vi "Build_from_Wizard.vi"(8 "error in (no error)":errorcluster, 9 "programmatic":bool, 10 "preview":bool, 11 "Class in":refnum<class "Installer.lvclass">) -> (0 "error out":errorcluster, 3 "Class out":refnum<class "Installer.lvclass">)   [LabVIEW 2020, in "Installer.lvclass"]
uses:
  <vilib>/AppBuilder/IB_Classes/Installer/Installer.lvclass
  <vilib>/AppBuilder/IB_Classes/Installer/Installer.lvclass/Installer.ctl
  <resource>/Framework/Providers/API/mxLvBuildError.ctl
  <resource>/Framework/Providers/Common/provcom_ProgressBar_Events.ctl
  <resource>/Framework/Providers/Common/provcom_StringGlobals.vi
  <resource>/Framework/Providers/Common/provcom_ProgressBar_Dialog_Text.ctl
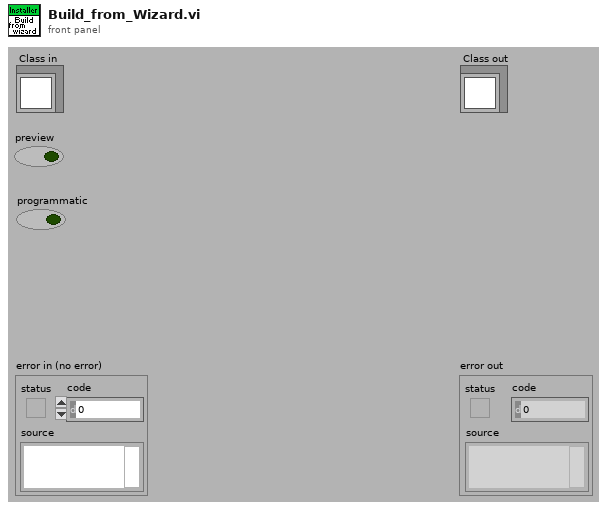
[diagram p1: front panel]
types:
  T1 = typedef "provcom_ProgressBar_Events.ctl" = cluster{"newJob":refnum<user-event>, "newItem":refnum<user-event>, "errorMsg":T2, "cancel":refnum<user-event>}
  T2 = typedef "mxLvBuildError.ctl" = refnum<user-event>
  T3 = typedef "provcom_ProgressBar_Dialog_Text.ctl" = cluster{"Operation action label":string, "Window title":string, "Expand text":string}
  T4 = typedef "mxLvBuildNewJob.ctl" = refnum<user-event>
  T5 = typedef "mxLvBuildNewItem.ctl" = refnum<user-event>
  T6 = typedef "mxLvBuildCancel.ctl" = refnum<user-event>
  T7 = typedef "ItemRef.ctl" = u64
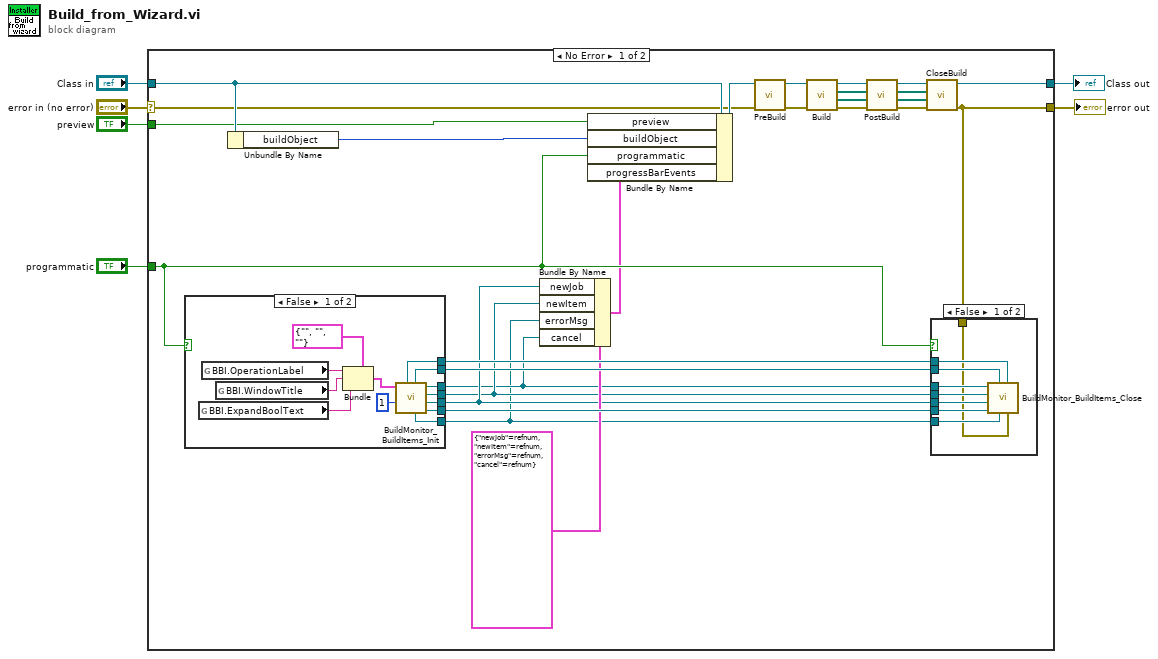
[diagram p0: block diagram]
diagram:
  n1 = case shown="No Error" "error in (no error)" {
    selector: "error in (no error)" -> [w7 w56]
    tunnel: [w14 w56] -> w5
    tunnel: [w20 w55] -> w3
    tunnel: "Class in" -> [w30 w55]
    tunnel: "preview" -> [w10 _]
    tunnel: "programmatic" -> [w9 _]
    frame No Error {
      n2 = case shown="False" w9 {
        tunnel: [w54 _] -> w33
        tunnel: [w53 _] -> w32
        tunnel: [w52 _] -> w31
        tunnel: [w51 _] -> w16
        tunnel: [w50 _] -> w17
        tunnel: [w49 _] -> w18
        tunnel: [w48 _] -> w15
        frame False {
          n3 = global read "provcom_StringGlobals.vi" "BBI.ExpandBoolText"() -> (w42:string)
          n4 = global read "provcom_StringGlobals.vi" "BBI.OperationLabel"() -> (w44:string)
          n5 = global read "provcom_StringGlobals.vi" "BBI.WindowTitle"() -> (w43:string)
          n6 = Bundle(cluster=T3 {"Operation action label"="", "Window title"="", "Expand text"=""} ("progressBar_DialogText"), "Operation action label"=w44, "Window title"=w43, "Expand text"=w42) -> (w45:T3)
          n7 = call <resource>:"BuildMonitor_BuildItems_Init.vi"("NumOfJobs"=u16 1, "progressBar_DialogText"=w45) -> ("Complete"=w54:refnum<user-event>, "NewJob"=w49:T4, "NewItem"=w50:T5, "Cancel event"=w51:T6, "Error event"=w48:T2, "ErrorOpenEvent"=w53:refnum<user-event>, "ErrorCloseEvent"=w52:refnum<user-event>)  [unwired: 3 in]
        }
        frame True {
        }
      }
      n8 = Unbundle By Name(w30) -> ("buildObject"=w13:T7)
      n9 = Bundle By Name(cluster=T1 {"newJob"=refnum, "newItem"=refnum, "errorMsg"=refnum, "cancel"=refnum} ("progressBarEvents"), "newJob"=w18, "newItem"=w17, "errorMsg"=w15, "cancel"=w16) -> (w8:T1)
      n10 = Bundle By Name(cluster=w30, "preview"=w10, "buildObject"=w13, "programmatic"=w9, "progressBarEvents"=w8) -> (w21:refnum<class "Installer.lvclass">)
      n11 = call-dynamic "PreBuild.vi"("error in (no error)"=w7, "Class in"=w21) -> ("error out"=w23:errorcluster, "Class out"=w22:refnum<class "Installer.lvclass">)  [unwired: 8 out]
      n12 = call-dynamic "Build.vi"("error in (no error)"=w23, "Class in"=w22) -> ("error out"=w25:errorcluster, "GeneratedFiles out"=w11:path[], "GeneratedDirectories out"=w12:path[], "Class out"=w24:refnum<class "Installer.lvclass">)  [unwired: 6 out]
      n13 = call-dynamic "PostBuild.vi"("error in (no error)"=w25, "GeneratedFiles in"=w11, "GeneratedDirectories in"=w12, "Class in"=w24) -> ("error out"=w26:errorcluster, "GeneratedFiles out"=w28:path[], "GeneratedDirectories out"=w27:path[], "Class out"=w29:refnum<class "Installer.lvclass">)  [unwired: 4 out]
      n14 = call-dynamic "CloseBuild.vi"("error in (no error)"=w26, "GeneratedFiles"=w28, "GeneratedDirectories"=w27, "Class in"=w29) -> ("error out"=w14:errorcluster, "Class out"=w20:refnum<class "Installer.lvclass">)  [unwired: 6 out]
      n15 = case shown="False" w9 {
        tunnel: w33 -> [w41 _]
        tunnel: w32 -> [w40 _]
        tunnel: w31 -> [w39 _]
        tunnel: w16 -> [w38 _]
        tunnel: w17 -> [w37 _]
        tunnel: w18 -> [w36 _]
        tunnel: w15 -> [w35 _]
        tunnel: w14 -> [w34 _]
        frame False {
          n16 = call <resource>:"BuildMonitor_BuildItems_Close.vi"("error IO"=w34, "ErrorCloseEvent"=w39, "Error event"=w35, "ErrorOpenEvent"=w40, "Complete"=w41, "NewJob"=w36, "NewItem"=w37, "Cancel event"=w38) -> ()  [unwired: 1 in, 3 out]
        }
        frame True {
        }
      }
    }
    frame Error {
    }
  }
  "error out" <- w5
  "Class out" <- w3
